vi "Scaffold Folders.vi"(10 "INI Filename":string, 11 "Item Ref":T1) -> ()   [LabVIEW 2020, in "Negentropic IDE.lvlib"]
uses:
  Negentropic IDE.lvlib
  <resource>/Framework/Providers/API/ItemRef.ctl
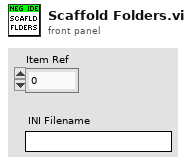
[diagram p1: front panel]
types:
  T1 = typedef "ItemRef.ctl" = u64
  T2 = typedef "Negentropic IDE.lvlib/Folder Config.ctl" = cluster{"Path":string, "Scope":T3}
  T3 = typedef "Negentropic IDE.lvlib/Scope.ctl" = enum32{"invalid scope", "public", "private", "protected", "community"}
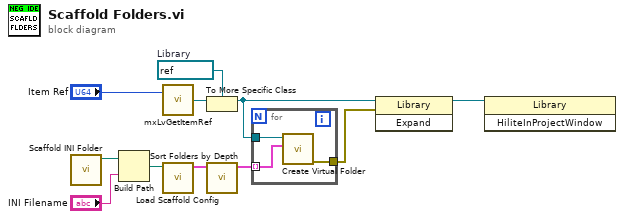
[diagram p0: block diagram]
diagram:
  w4 = refnum<vi> refnum  # Library
  n1 = call "Scaffold INI Folder.vi"() -> ("Scaffold INI Folder"=w9:path)  [unwired: 10 in, 1 out]
  n2 = Build Path(base path=w9, name or relative path="INI Filename") -> (appended path=w8:path)
  n3 = call <resource>:"mxLvGetItemRef.vi"("Item"="Item Ref") -> ("Item Refnum"=w5:refnum<vi>)  [unwired: 1 in, 2 out]
  n4 = call "Load Scaffold Config.vi"("Path"=w8) -> ("Folders"=w7:T2[])  [unwired: 9 in, 1 out]
  n5 = To More Specific Class(target class=w4, reference=w5) -> (specific class reference=w3:refnum<vi>)  [unwired: 1 in, 1 out]
  n6 = call "Sort Folders by Depth.vi"("Folders In"=w7) -> ("Sorted Folders"=w6:T2[])  [unwired: 10 in]
  n7 = for {
    tunnel: w6 -> [w13] mode=indexing
    tunnel: w3 -> [w14]
    tunnel: [w12] -> w2
    n8 = call "Create Virtual Folder.vi"("Folder Config"=w13, "Library"=w14) -> ("error out"=w12:errorcluster)  [unwired: 8 in, 1 out]
  }
  n9 = invoke class="Library" method="Expand"(reference=w3, error in=w2) -> (reference out=w1:refnum<vi>)  [unwired: 1 in, 2 out]
  n10 = invoke class="Library" method="HiliteInProjectWindow"(reference=w1) -> ()  [unwired: 2 in, 3 out]
